vi "Out_S6F1.vi"(8 "error in (no error)":errorcluster, 10 "S6F1":T1, 11 "S6 Message Class in":refnum<class "S6 Message Class.lvclass">) -> (0 "error out":errorcluster, 3 "S6 Message Class out":refnum<class "S6 Message Class.lvclass">)   [LabVIEW 2020, in "SECS Communication.lvlib" / "S6 Message Class.lvclass"]
uses:
  S6 Message Class.lvclass
  D:/Dropbox/SECS/SECS_GEM v1.0.6/Com/SECS Communication/SECS-II Class/SECS-II Class.lvclass
  S6F1.ctl
  SECS-II Class/Format Code.ctl
  SECS-II Class/Data Message_List.vi
  SECS-II Class/Data Message_U4.vi
  SECS-II Class/Data Message_ASCII.vi
  SECS-II Class/Variant To Data_ASCII.vi
  SECS-II Class/Variant To Data_Binary.vi
  SECS-II Class/Data Message_Binary.vi
  SECS-II Class/Variant To Data_Boolean.vi
  SECS-II Class/Data Message_Boolean.vi
  SECS-II Class/Variant To Data_J.vi
  SECS-II Class/Data Message_J.vi
  SECS-II Class/Variant To Data_I1.vi
  SECS-II Class/Data Message_I1 .vi
  SECS-II Class/Variant To Data_I2.vi
  SECS-II Class/Data Message_I2.vi
  SECS-II Class/Variant To Data_I4.vi
  SECS-II Class/Data Message_I4.vi
  SECS-II Class/Variant To Data_I8.vi
  SECS-II Class/Data Message_I8.vi
  SECS-II Class/Variant To Data_U1.vi
  SECS-II Class/Data Message_U1.vi
  SECS-II Class/Variant To Data_U2.vi
  SECS-II Class/Data Message_U2.vi
  SECS-II Class/Variant To Data_U4.vi
  SECS-II Class/Variant To Data_U8.vi
  SECS-II Class/Data Message_U8.vi
  SECS-II Class/Variant To Data_F4.vi
  SECS-II Class/Data Message_F4.vi
  SECS-II Class/Variant To Data_F8.vi
  SECS-II Class/Data Message_F8.vi
  SECS-II Class/Variant To Data_Character.vi
  SECS-II Class/Data Message_Character.vi
  SECS-II Class/SECS-II Class.lvclass
  D:/Dropbox/SECS/SECS_GEM v1.0.6/Com/SECS Communication/S6 Message Class/S6 Message Class.lvclass
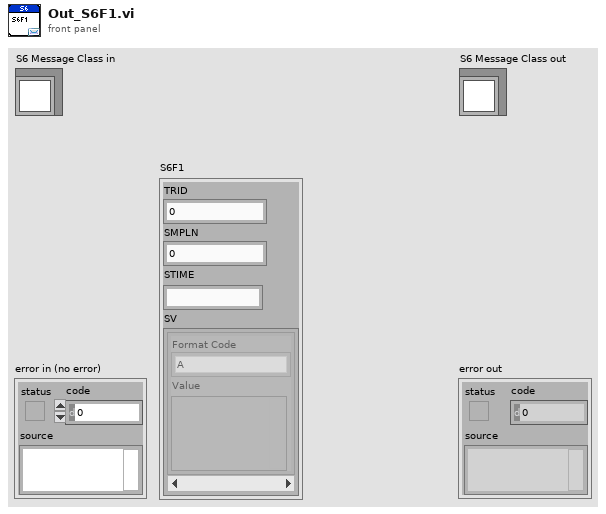
[diagram p1: front panel]
types:
  T1 = typedef "SECS Communication.lvlib/S6 Message Class.lvclass/S6F1.ctl" = cluster{"TRID":u32, "SMPLN":u32, "STIME":string, "SV":cluster{"Format Code":T2, "Value":variant}[]}
  T2 = typedef "SECS Communication.lvlib/SECS-II Class.lvclass/Format Code.ctl" = enum16{"L", "A", "B", "Boolean", "J", "I1", "I2", "I4", "I8", "U1", "U2", "U4", "U8", "F4", "F8", "Char"}
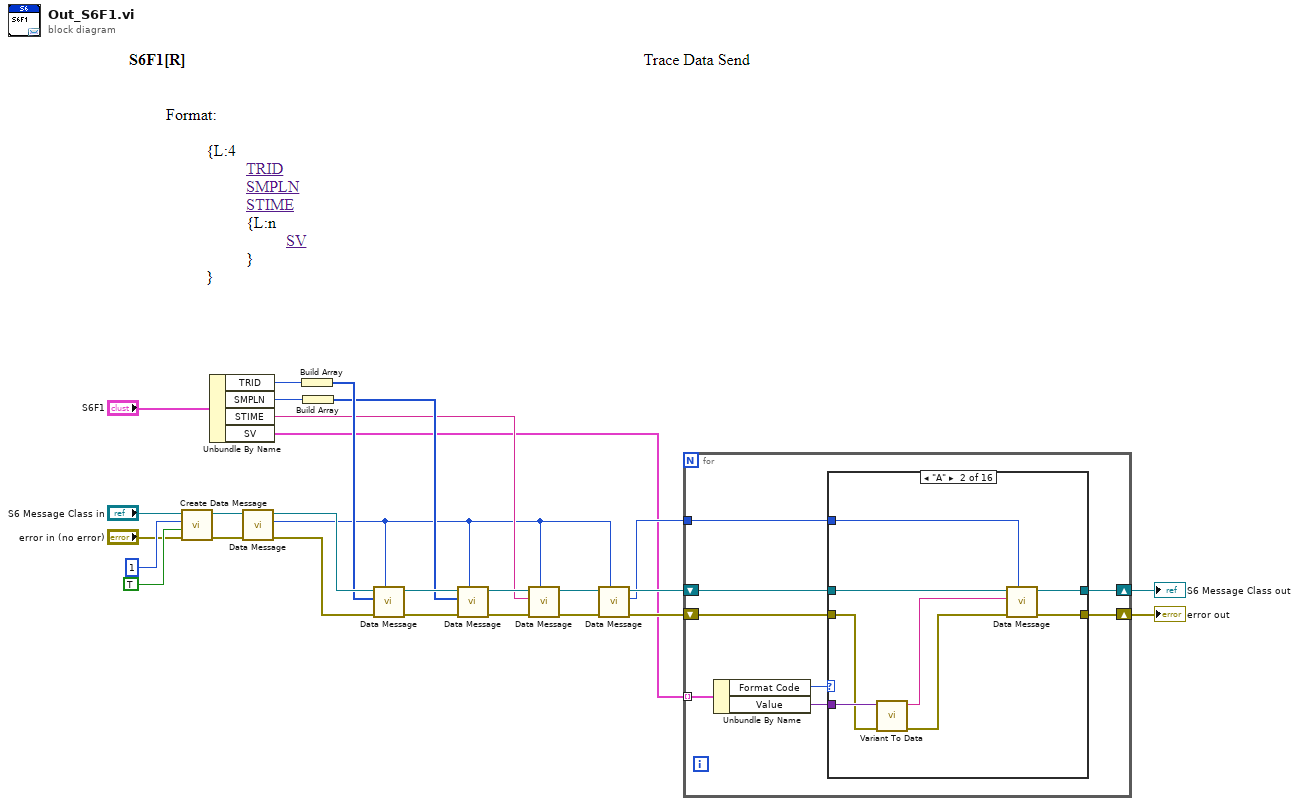
[diagram p0: block diagram]
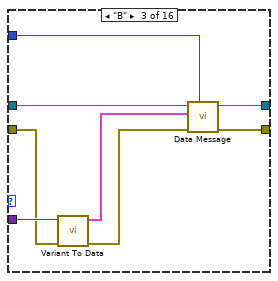
[diagram p3: hidden frame]
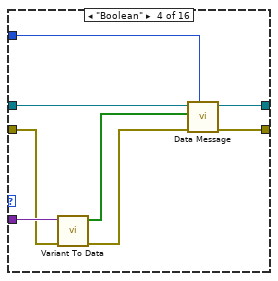
[diagram p4: hidden frame]
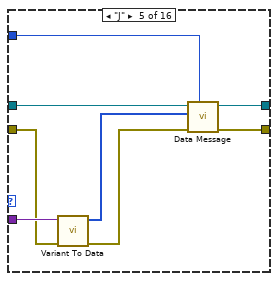
[diagram p5: hidden frame]
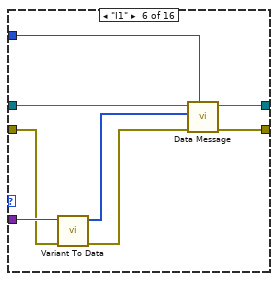
[diagram p6: hidden frame]
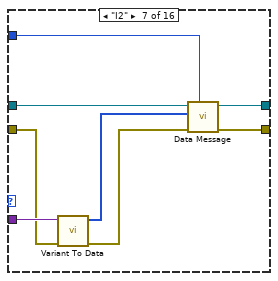
[diagram p7: hidden frame]
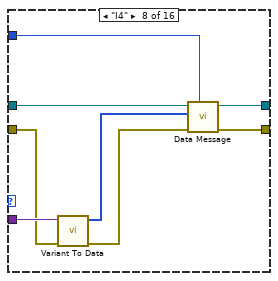
[diagram p8: hidden frame]
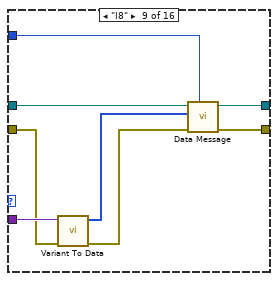
[diagram p9: hidden frame]
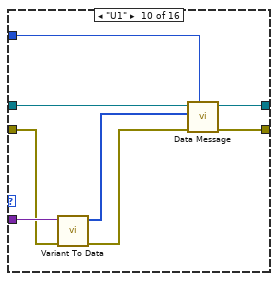
[diagram p10: hidden frame]
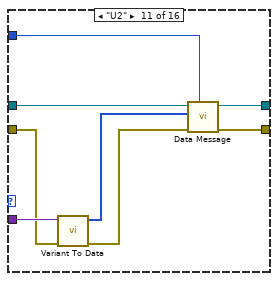
[diagram p11: hidden frame]
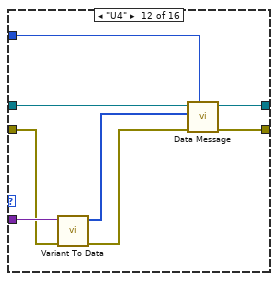
[diagram p12: hidden frame]
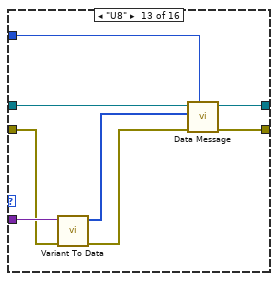
[diagram p13: hidden frame]
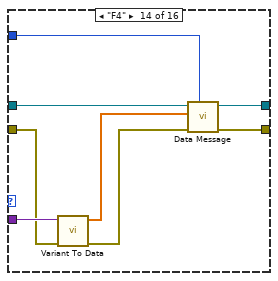
[diagram p14: hidden frame]
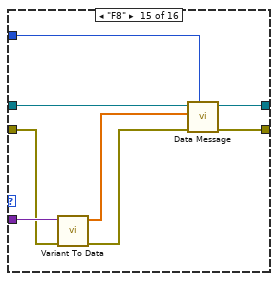
[diagram p15: hidden frame]
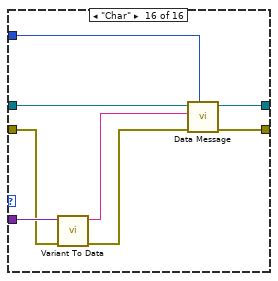
[diagram p16: hidden frame]
diagram:
  n1 = call "Create Data Message.vi"("error in (no error)"="error in (no error)", "W-Bit"=TRUE, "Function"=u8 1, "SECS-II Class in"="S6 Message Class in") -> ("error out"=w24:errorcluster, "SECS-II Class out"=w25:refnum<class "S6 Message Class.lvclass">)  [unwired: 6 in]
  n2 = Unbundle By Name("S6F1") -> ("TRID"=w19:u32, "SMPLN"=w15:u32, "STIME"=w10:string, "SV"=w3:cluster{"Format Code":T2, "Value":variant}[])
  n3 = call-poly "Data Message.vi"("error in"=w24, "SECS-II Class in"=w25) -> ("error out"=w20:errorcluster, "Index"=w7:i32, "SECS-II Class out"=w21:refnum<class "S6 Message Class.lvclass">)  [unwired: 7 in]
  n4 = Build Array(w19) -> (w18:u32[])
  n5 = Build Array(w15) -> (w14:u32[])
  n6 = call-poly "Data Message.vi"("Parent Index"=w7, "error in"=w20, "Data"=w18, "SECS-II Class in"=w21) -> ("error out"=w16:errorcluster, "SECS-II Class out"=w17:refnum<class "S6 Message Class.lvclass">)  [unwired: 6 in]
  n7 = call-poly "Data Message.vi"("Parent Index"=w7, "error in"=w16, "Data"=w14, "SECS-II Class in"=w17) -> ("error out"=w12:errorcluster, "SECS-II Class out"=w11:refnum<class "S6 Message Class.lvclass">)  [unwired: 6 in]
  n8 = call-poly "Data Message.vi"("Parent Index"=w7, "error in"=w12, "Data"=w10, "SECS-II Class in"=w11) -> ("error out"=w8:errorcluster, "SECS-II Class out"=w9:refnum<class "S6 Message Class.lvclass">)  [unwired: 6 in]
  n9 = call-poly "Data Message.vi"("Parent Index"=w7, "error in"=w8, "SECS-II Class in"=w9) -> ("error out"=w5:errorcluster, "Index"=w4:i32, "SECS-II Class out"=w6:refnum<class "S6 Message Class.lvclass">)  [unwired: 6 in]
  n10 = for {
    shift-right: [w31] -> w1
    shift-left: w5 -> [w28]
    shift-right: [w32] -> w2
    shift-left: w6 -> [w29]
    tunnel: w3 -> [w35] mode=indexing
    tunnel: w4 -> [w30]
    n11 = Unbundle By Name(w35) -> ("Format Code"=w34:T2, "Value"=w33:variant)
    n12 = case shown="\"A\"" w34 {
      tunnel: w33 -> [_ w41 w49 w57 w65 w73 w81 w89 w97 w105 w113 w121 w129 w137 w145 w153]
      tunnel: w29 -> [w37 w45 w53 w61 w69 w77 w85 w93 w101 w109 w117 w125 w133 w141 w149 w157]
      tunnel: w28 -> [w36 w40 w48 w56 w64 w72 w80 w88 w96 w104 w112 w120 w128 w136 w144 w152]
      tunnel: [w37 w43 w51 w59 w67 w75 w83 w91 w99 w107 w115 w123 w131 w139 w147 w155] -> w32
      tunnel: [w36 w42 w50 w58 w66 w74 w82 w90 w98 w106 w114 w122 w130 w138 w146 w154] -> w31
      tunnel: w30 -> [_ w44 w52 w60 w68 w76 w84 w92 w100 w108 w116 w124 w132 w140 w148 w156]
      frame "L", Default {
      }
      frame "A" {
        n13 = call-poly "Variant To Data.vi"("error in (no error)"=w40, "Variant"=w41) -> ("error out"=w39:errorcluster, "Data"=w38:string)  [unwired: 7 in, 1 out]
        n14 = call-poly "Data Message.vi"("Parent Index"=w44, "error in"=w39, "Data"=w38, "SECS-II Class in"=w45) -> ("error out"=w42:errorcluster, "SECS-II Class out"=w43:refnum<class "S6 Message Class.lvclass">)  [unwired: 6 in]
      }
      frame "B" {
        n15 = call-poly "Variant To Data.vi"("error in (no error)"=w48, "Variant"=w49) -> ("error out"=w47:errorcluster, "Data Cluster"=w46:cluster{"Data":bool[]}[])  [unwired: 7 in, 1 out]
        n16 = call-poly "Data Message.vi"("Parent Index"=w52, "error in"=w47, "Data Cluster"=w46, "SECS-II Class in"=w53) -> ("error out"=w50:errorcluster, "SECS-II Class out"=w51:refnum<class "S6 Message Class.lvclass">)  [unwired: 6 in]
      }
      frame "Boolean" {
        n17 = call-poly "Variant To Data.vi"("error in (no error)"=w56, "Variant"=w57) -> ("error out"=w55:errorcluster, "Data"=w54:bool[])  [unwired: 7 in, 1 out]
        n18 = call-poly "Data Message.vi"("Parent Index"=w60, "error in"=w55, "Data"=w54, "SECS-II Class in"=w61) -> ("error out"=w58:errorcluster, "SECS-II Class out"=w59:refnum<class "S6 Message Class.lvclass">)  [unwired: 6 in]
      }
      frame "J" {
        n19 = call-poly "Variant To Data.vi"("error in (no error)"=w64, "Variant"=w65) -> ("error out"=w63:errorcluster, "Data"=w62:i64[])  [unwired: 7 in, 1 out]
        n20 = call-poly "Data Message.vi"("Parent Index"=w68, "error in"=w63, "Data"=w62, "SECS-II Class in"=w69) -> ("error out"=w66:errorcluster, "SECS-II Class out"=w67:refnum<class "S6 Message Class.lvclass">)  [unwired: 6 in]
      }
      frame "I1" {
        n21 = call-poly "Variant To Data.vi"("error in (no error)"=w72, "Variant"=w73) -> ("error out"=w71:errorcluster, "Data"=w70:i8[])  [unwired: 7 in, 1 out]
        n22 = call-poly "Data Message.vi"("Parent Index"=w76, "error in"=w71, "Data"=w70, "SECS-II Class in"=w77) -> ("error out"=w74:errorcluster, "SECS-II Class out"=w75:refnum<class "S6 Message Class.lvclass">)  [unwired: 6 in]
      }
      frame "I2" {
        n23 = call-poly "Variant To Data.vi"("error in (no error)"=w80, "Variant"=w81) -> ("error out"=w79:errorcluster, "Data"=w78:i16[])  [unwired: 7 in, 1 out]
        n24 = call-poly "Data Message.vi"("Parent Index"=w84, "error in"=w79, "Data"=w78, "SECS-II Class in"=w85) -> ("error out"=w82:errorcluster, "SECS-II Class out"=w83:refnum<class "S6 Message Class.lvclass">)  [unwired: 6 in]
      }
      frame "I4" {
        n25 = call-poly "Variant To Data.vi"("error in (no error)"=w88, "Variant"=w89) -> ("error out"=w87:errorcluster, "Data"=w86:i32[])  [unwired: 7 in, 1 out]
        n26 = call-poly "Data Message.vi"("Parent Index"=w92, "error in"=w87, "Data"=w86, "SECS-II Class in"=w93) -> ("error out"=w90:errorcluster, "SECS-II Class out"=w91:refnum<class "S6 Message Class.lvclass">)  [unwired: 6 in]
      }
      frame "I8" {
        n27 = call-poly "Variant To Data.vi"("error in (no error)"=w96, "Variant"=w97) -> ("error out"=w95:errorcluster, "Data"=w94:i64[])  [unwired: 7 in, 1 out]
        n28 = call-poly "Data Message.vi"("Parent Index"=w100, "error in"=w95, "Data"=w94, "SECS-II Class in"=w101) -> ("error out"=w98:errorcluster, "SECS-II Class out"=w99:refnum<class "S6 Message Class.lvclass">)  [unwired: 6 in]
      }
      frame "U1" {
        n29 = call-poly "Variant To Data.vi"("error in (no error)"=w104, "Variant"=w105) -> ("error out"=w103:errorcluster, "Data"=w102:u8[])  [unwired: 7 in, 1 out]
        n30 = call-poly "Data Message.vi"("Parent Index"=w108, "error in"=w103, "Data"=w102, "SECS-II Class in"=w109) -> ("error out"=w106:errorcluster, "SECS-II Class out"=w107:refnum<class "S6 Message Class.lvclass">)  [unwired: 6 in]
      }
      frame "U2" {
        n31 = call-poly "Variant To Data.vi"("error in (no error)"=w112, "Variant"=w113) -> ("error out"=w111:errorcluster, "Data"=w110:u16[])  [unwired: 7 in, 1 out]
        n32 = call-poly "Data Message.vi"("Parent Index"=w116, "error in"=w111, "Data"=w110, "SECS-II Class in"=w117) -> ("error out"=w114:errorcluster, "SECS-II Class out"=w115:refnum<class "S6 Message Class.lvclass">)  [unwired: 6 in]
      }
      frame "U4" {
        n33 = call-poly "Variant To Data.vi"("error in (no error)"=w120, "Variant"=w121) -> ("error out"=w119:errorcluster, "Data"=w118:u32[])  [unwired: 7 in, 1 out]
        n34 = call-poly "Data Message.vi"("Parent Index"=w124, "error in"=w119, "Data"=w118, "SECS-II Class in"=w125) -> ("error out"=w122:errorcluster, "SECS-II Class out"=w123:refnum<class "S6 Message Class.lvclass">)  [unwired: 6 in]
      }
      frame "U8" {
        n35 = call-poly "Variant To Data.vi"("error in (no error)"=w128, "Variant"=w129) -> ("error out"=w127:errorcluster, "Data"=w126:u64[])  [unwired: 7 in, 1 out]
        n36 = call-poly "Data Message.vi"("Parent Index"=w132, "error in"=w127, "Data"=w126, "SECS-II Class in"=w133) -> ("error out"=w130:errorcluster, "SECS-II Class out"=w131:refnum<class "S6 Message Class.lvclass">)  [unwired: 6 in]
      }
      frame "F4" {
        n37 = call-poly "Variant To Data.vi"("error in (no error)"=w136, "Variant"=w137) -> ("error out"=w135:errorcluster, "Data"=w134:sgl[])  [unwired: 7 in, 1 out]
        n38 = call-poly "Data Message.vi"("Parent Index"=w140, "error in"=w135, "Data"=w134, "SECS-II Class in"=w141) -> ("error out"=w138:errorcluster, "SECS-II Class out"=w139:refnum<class "S6 Message Class.lvclass">)  [unwired: 6 in]
      }
      frame "F8" {
        n39 = call-poly "Variant To Data.vi"("error in (no error)"=w144, "Variant"=w145) -> ("error out"=w143:errorcluster, "Data"=w142:dbl[])  [unwired: 7 in, 1 out]
        n40 = call-poly "Data Message.vi"("Parent Index"=w148, "error in"=w143, "Data"=w142, "SECS-II Class in"=w149) -> ("error out"=w146:errorcluster, "SECS-II Class out"=w147:refnum<class "S6 Message Class.lvclass">)  [unwired: 6 in]
      }
      frame "Char" {
        n41 = call-poly "Variant To Data.vi"("error in (no error)"=w152, "Variant"=w153) -> ("error out"=w151:errorcluster, "Data"=w150:string)  [unwired: 7 in, 1 out]
        n42 = call-poly "Data Message.vi"("Parent Index"=w156, "error in"=w151, "Data"=w150, "SECS-II Class in"=w157) -> ("error out"=w154:errorcluster, "SECS-II Class out"=w155:refnum<class "S6 Message Class.lvclass">)  [unwired: 6 in]
      }
    }
  }
  "error out" <- w1
  "S6 Message Class out" <- w2
